vi "InitializeKeithley6482.vi"(8 "Error In":errorcluster, 10 "Keithley 6482":T1, 11 "VISA Resources":string[](array[string])) -> (0 "Error Out":errorcluster, 3 "Keithley 6482 Out":refnum<visa-resource-name>[](array[refnum]))   [LabVIEW 2012]
uses:
  Keithley6482Configuration.ctl
  libs/Keithley-6482/Public/Controls/DataFormat.ctl
  libs/Keithley-6482/Keithley-6482.lvlib
  libs/LV-Utilities/LV-Utilities.lvlib
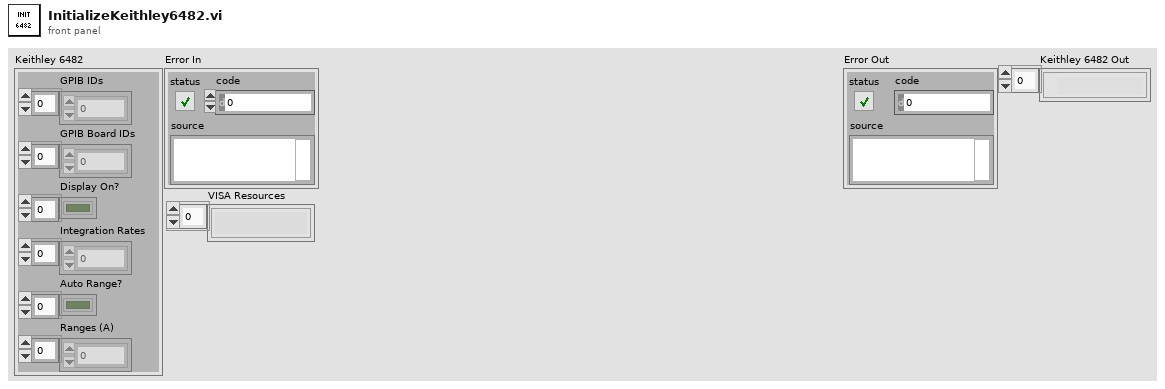
[diagram p1: front panel]
types:
  T1 = typedef "Keithley6482Configuration.ctl" = cluster{"GPIB IDs":u8[], "GPIB Board IDs":u8[], "Display On?":bool[], "Integration Rates":dbl[], "Auto Range?":bool[], "Ranges (A)":dbl[]}
  T2 = typedef "Keithley-6482.lvlib/DataFormat.ctl" = enum16{"ASCII", "Real", "32", "Sreal"}
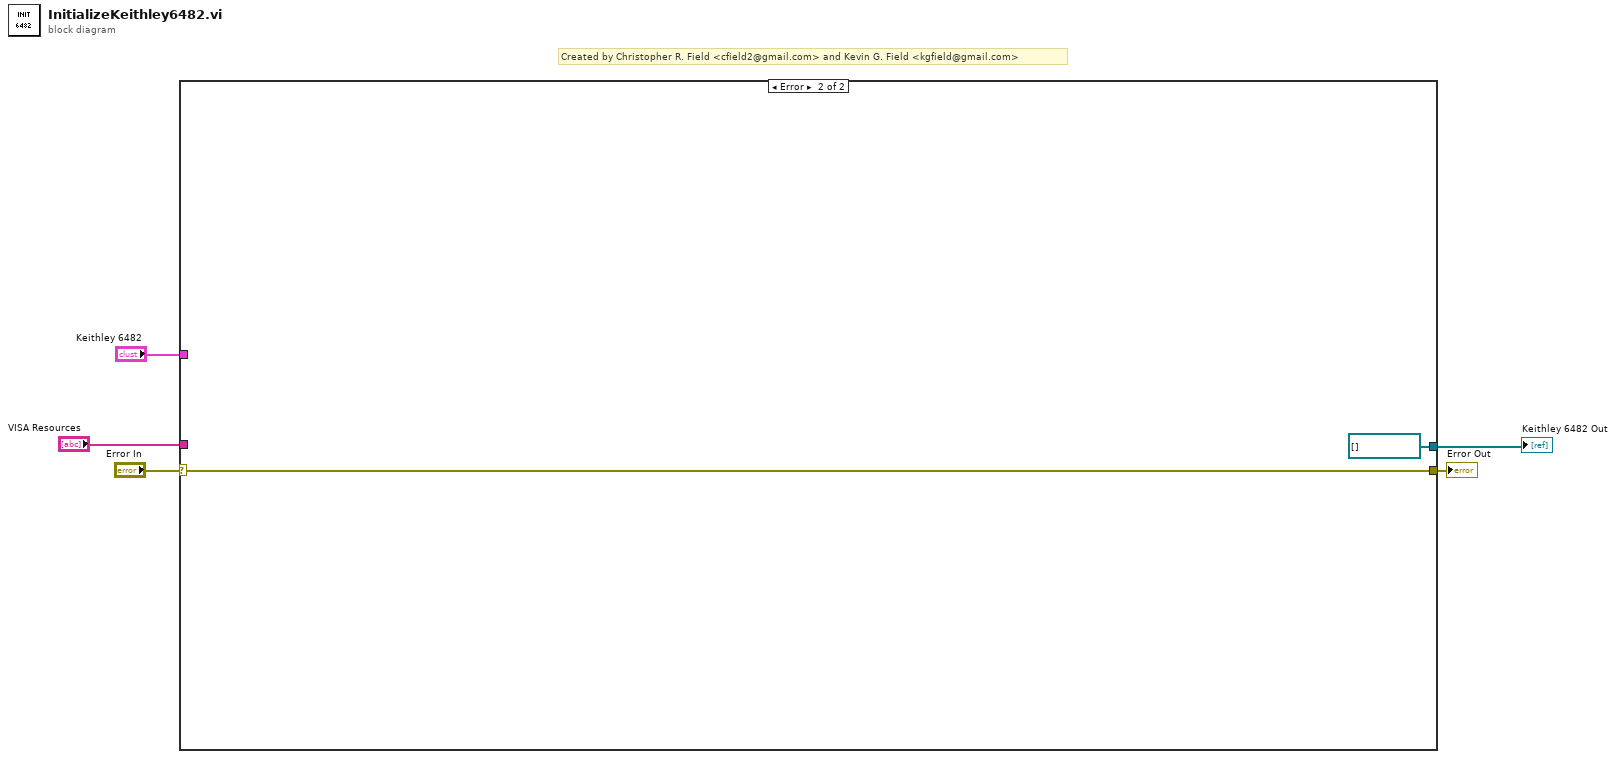
[diagram p0: block diagram]
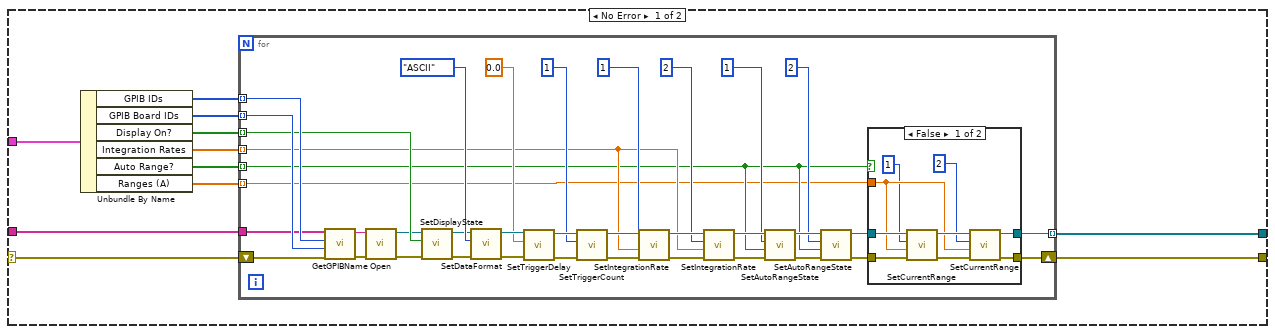
[diagram p2: hidden frame]
diagram:
  # "Created by Christopher R. Field <cfield2@gmail.com> and Kevin G. Field <kgfield@gmail.com>"
  n1 = case shown="Error" "Error In" {
    selector: "Error In" -> [w7 w66]
    tunnel: "Keithley 6482" -> [w10 _]
    tunnel: [w9 w66] -> w4
    tunnel: [w8 refnum<visa-resource-name>[] []] -> w3
    tunnel: "VISA Resources" -> [w6 _]
    frame No Error {
      n2 = Unbundle By Name(w10) -> ("GPIB IDs"=w16:u8[], "GPIB Board IDs"=w15:u8[], "Display On?"=w14:bool[], "Integration Rates"=w13:dbl[], "Auto Range?"=w12:bool[], "Ranges (A)"=w11:dbl[])
      n3 = for {
        tunnel: w16 -> [w53] mode=indexing
        tunnel: w15 -> [w52] mode=indexing
        tunnel: w14 -> [w49] mode=indexing
        tunnel: [w19] -> w8 mode=indexing
        shift-right: [w20] -> w9
        shift-left: w7 -> [w25]
        tunnel: w13 -> [w24] mode=indexing
        tunnel: w12 -> [w22] mode=indexing
        tunnel: w11 -> [w18] mode=indexing
        tunnel: w6 -> [w17]
        n4 = call "GetGPIBName.vi"("Error In"=w25, "GPIB ID"=w52, "GPIB Board"=w53, "VISA Resource List"=w17) -> ("Error Out"=w50:errorcluster, "VISA GPIB Resource Name"=w51:string)  [unwired: 5 in, 1 out]
        n5 = call "Open.vi"("Error In"=w50, "Keithley 6482 In"=w51) -> ("Error Out"=w47:errorcluster, "Keithley 6482 Out"=w48:refnum<visa-resource-name>)  [unwired: 8 in]
        n6 = call "SetDisplayState.vi"("Error In"=w47, "Enabled?"=w49, "Keithley 6482 In"=w48) -> ("Error Out"=w38:errorcluster, "Keithley 6482 Out"=w39:refnum<visa-resource-name>)  [unwired: 7 in]
        n7 = call "SetDataFormat.vi"("Error In"=w38, "Data Format"=DataFormat."ASCII", "Keithley 6482 In"=w39) -> ("Error Out"=w44:errorcluster, "Keithley 6482 Out"=w45:refnum<visa-resource-name>)  [unwired: 7 in]
        n8 = call "SetTriggerDelay.vi"("Error In"=w44, "Delay (sec)"=0.0, "Keithley 6482 In"=w45) -> ("Error Out"=w41:errorcluster, "Keithley 6482 Out"=w42:refnum<visa-resource-name>)  [unwired: 7 in]
        n9 = call "SetTriggerCount.vi"("Error In"=w41, "Count (1-3000)"=u16 1, "Keithley 6482 In"=w42) -> ("Error Out"=w36:errorcluster, "Keithley 6482 Out"=w37:refnum<visa-resource-name>)  [unwired: 7 in]
        n10 = call "SetIntegrationRate.vi"("Error In"=w36, "Integration Rate"=w24, "Channel (1 or 2)"=u8 1, "Keithley 6482 In"=w37) -> ("Error Out"=w33:errorcluster, "Keithley 6482 Out"=w34:refnum<visa-resource-name>)  [unwired: 6 in]
        n11 = call "SetIntegrationRate.vi"("Error In"=w33, "Integration Rate"=w24, "Channel (1 or 2)"=u8 2, "Keithley 6482 In"=w34) -> ("Error Out"=w30:errorcluster, "Keithley 6482 Out"=w31:refnum<visa-resource-name>)  [unwired: 6 in]
        n12 = call "SetAutoRangeState.vi"("Error In"=w30, "Enabled?"=w22, "Channel (1 or 2)"=u8 1, "Keithley 6482 In"=w31) -> ("Error Out"=w27:errorcluster, "Keithley 6482 Out"=w28:refnum<visa-resource-name>)  [unwired: 6 in]
        n13 = call "SetAutoRangeState.vi"("Error In"=w27, "Enabled?"=w22, "Channel (1 or 2)"=u8 2, "Keithley 6482 In"=w28) -> ("Error Out"=w23:errorcluster, "Keithley 6482 Out"=w21:refnum<visa-resource-name>)  [unwired: 6 in]
        n14 = case shown="False" w22 {
          tunnel: w23 -> [w57 w64]
          tunnel: w21 -> [w62 w63]
          tunnel: [w59 w64] -> w20
          tunnel: [w60 w63] -> w19
          tunnel: w18 -> [w56 _]
          frame False {
            n15 = call "SetCurrentRange.vi"("Error In"=w57, "Expected Current (A)"=w56, "Channel (1 or 2)"=u8 1, "Keithley 6482 In"=w62) -> ("Error Out"=w58:errorcluster, "Keithley 6482 Out"=w61:refnum<visa-resource-name>)  [unwired: 6 in]
            n16 = call "SetCurrentRange.vi"("Error In"=w58, "Expected Current (A)"=w56, "Channel (1 or 2)"=u8 2, "Keithley 6482 In"=w61) -> ("Error Out"=w59:errorcluster, "Keithley 6482 Out"=w60:refnum<visa-resource-name>)  [unwired: 6 in]
          }
          frame True {
          }
        }
      }
    }
    frame Error {
    }
  }
  "Error Out" <- w4
  "Keithley 6482 Out" <- w3
